vi "registerDataEvent.vi"(8 "error in (no error)":errorcluster, 9 "Callback VI Ref":refnum<vi>, 10 "Event Callback in":refnum<k27>, 11 "SM1000-control in":T1) -> (0 "error out":errorcluster, 2 "Event Callback":refnum<k27>, 3 "SM1000-control out":T1)   [LabVIEW 2013, in "HardwareCharacterization.lvlib" / "HC-SM1000.lvclass"]
doc: "Registers for application and exception events returned from the EC device session.\nThe method 'handleConnectEvent' is called when the event is detected."
uses:
  HC-SM1000.lvclass
  Object-reference.ctl
  HC-SM1000.lvclass/HC-SM1000.ctl
  Custom-errors.ctl
  C:/Users/vangeste/Desktop/2015-05-29 - SLM - MAIF/HC-HardwareCharacterization/Sources/SM1000/LECSession.dll
  LECSession.dll
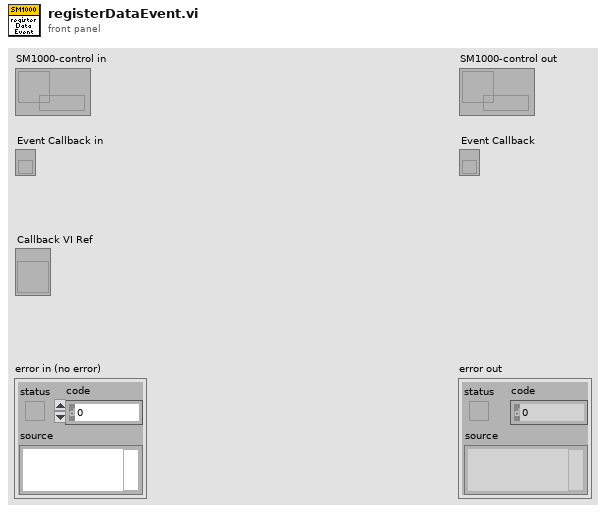
[diagram p1: front panel]
types:
  T1 = typedef "HardwareCharacterization.lvlib/HC-SM1000.lvclass/Object-reference.ctl" = refnum<data-value>
  T2 = typedef "HardwareCharacterization.lvlib/HC-SM1000.lvclass/Custom-errors.ctl" = enum16{"No error", "Not implemented", "Command not recognized", "Invalid input", "No connection", "Timeout", "Resource not loaded"}
  T3 = cluster{"puiPayloadHigh":u32, "puiPayloadLow":u32, "pstrData":string}
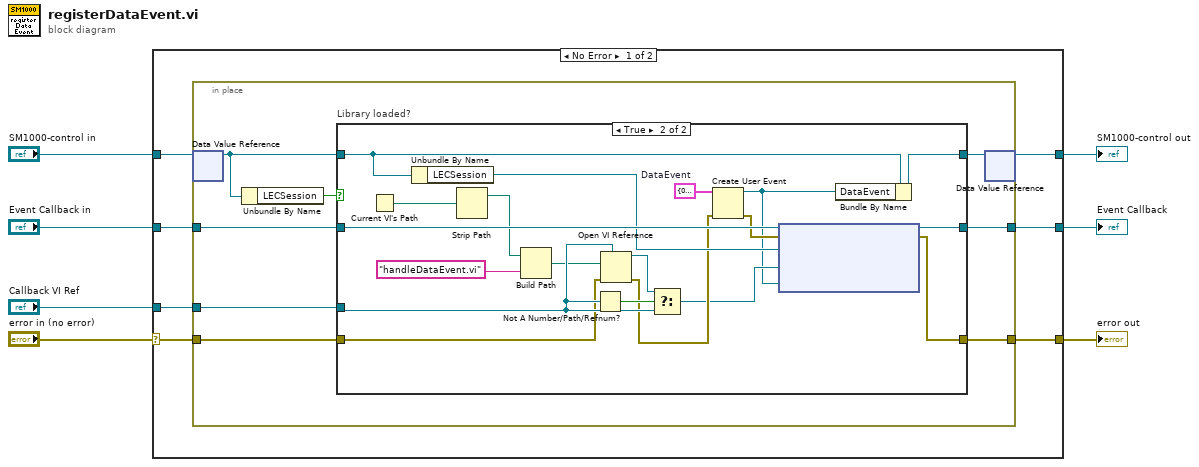
[diagram p0: block diagram]
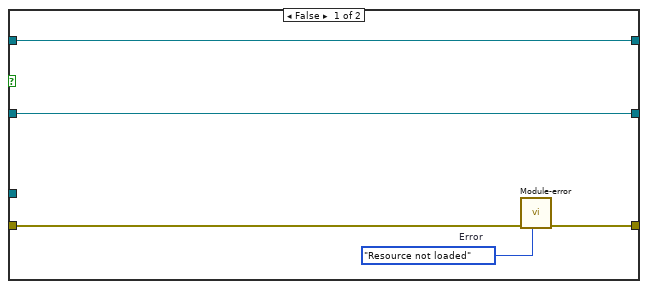
[diagram p2: hidden frame]
diagram:
  n1 = case shown="No Error" "error in (no error)" {
    selector: "error in (no error)" -> [w13 w49]
    tunnel: [w12 w49] -> w6
    tunnel: [w14 w48] -> w4
    tunnel: "SM1000-control in" -> [w8 w48]
    tunnel: "Event Callback in" -> [w11 w47]
    tunnel: "Callback VI Ref" -> [w10 _]
    tunnel: [w9 w47] -> w2
    frame No Error {
      n2 = in-place {
        in-place-border: w13 -> [w22]
        in-place-border: [w19] -> w12
        in-place-border: w11 -> [w17]
        in-place-border: w10 -> [w15]
        in-place-border: [w16] -> w9
        n3 = in-place-dvr #1(w8) -> (w20:refnum<class "HC-SM1000.lvclass">)  [unwired: 1 out]
        n4 = Unbundle By Name(w20) -> ("LECSession"=w21:bool)
        n5 = case "Library loaded?" shown="True" w21 {
          tunnel: w22 -> [w27 w38]
          tunnel: w20 -> [w25 w46]
          tunnel: [w26 w31] -> w19
          tunnel: [w25 w34] -> w18
          tunnel: w17 -> [w24 w45]
          tunnel: w15 -> [_ w41]
          tunnel: [w24 w44] -> w16
          frame False {
            w23 = Custom-errors."Resource not loaded"  # Error
            n6 = call "Module-error.vi"("Error"=w23, "error in (no error)"=w27) -> ("error out"=w26:errorcluster)  [unwired: 9 in]
          }
          frame True {
            w30 = T3 {"puiPayloadHigh"=0, "puiPayloadLow"=0, "pstrData"=""}  # DataEvent
            n7 = Current VI's Path() -> (path=w36:path)
            n8 = Unbundle By Name(w46) -> ("LECSession"=w43:refnum<k24>)
            n9 = Strip Path(path=w36) -> (stripped path=w35:path)  [unwired: 1 out]
            n10 = Build Path(base path=w35, name or relative path="handleDataEvent.vi") -> (appended path=w39:path)
            n11 = Not A Number/Path/Refnum?(number/path/refnum=w41) -> (NaN/Path/Refnum?=w42:bool)
            n12 = Open VI Reference(type specifier VI Refnum (for type only)=w41, vi path=w39, error in (no error)=w38) -> (vi reference=w37:refnum<vi>, error out=w33:errorcluster)  [unwired: 3 in]
            n13 = Select(t=w37, s=w42, f=w41) -> (s? t:f=w29:refnum<vi>)
            n14 = Create User Event(user event datatype=w30, error in=w33) -> (user event=w28:refnum<user-event>, error out=w32:errorcluster)
            n15 = node(w45, w32, w43, w29, w28) -> (w44:refnum<k27>, w31:errorcluster)
            n16 = Bundle By Name(cluster=w46, "DataEvent"=w28) -> (w34:refnum<class "HC-SM1000.lvclass">)
          }
        }
        n17 = in-place-dvr #1(w18) -> (w14:T1)  [unwired: 1 out]
      }
    }
    frame Error {
    }
  }
  "error out" <- w6
  "SM1000-control out" <- w4
  "Event Callback" <- w2
